vi "Write Timings Header.vi"(8 "error in (no error)":errorcluster, 11 "Save Image in":refnum<class "Save Image.lvclass">) -> (0 "error out":errorcluster, 3 "Save Image out":refnum<class "Save Image.lvclass">)   [LabVIEW 2018, in "Save Image.lvclass"]
uses:
  Save Image.lvclass
  <userlib>/gfitsio/gfitsio-write-key-string.vi
  <userlib>/gfitsio/gfitsio.lvlib
  Simulated_Header/Simulated_Header.lvclass
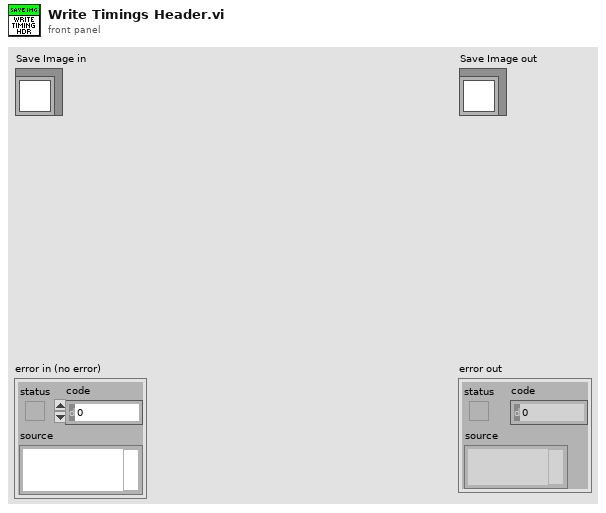
[diagram p1: front panel]
types:
  T1 = typedef "gfitsio.lvlib/gfitsio-refnum.ctl" = refnum<k1>
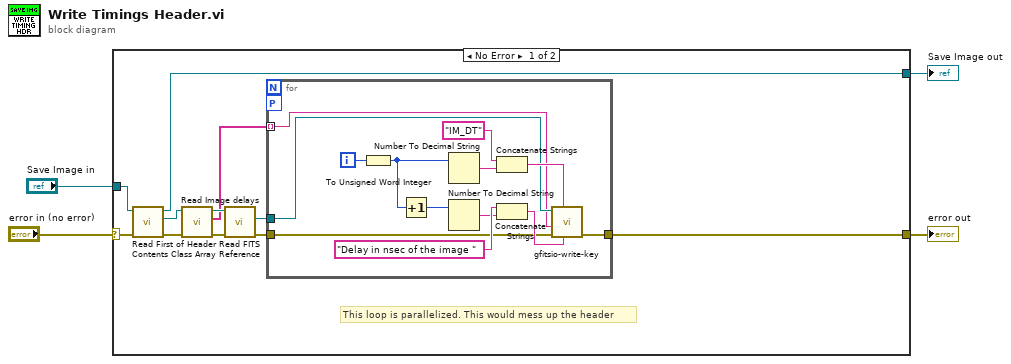
[diagram p0: block diagram]
diagram:
  n1 = case shown="No Error" "error in (no error)" {
    selector: "error in (no error)" -> [w11 w30]
    tunnel: [w15 w30] -> w3
    tunnel: [w5 w29] -> w1
    tunnel: "Save Image in" -> [w13 w29]
    frame No Error {
      # "This loop is parallelized. This would mess up the header"
      n2 = call "Read First of Header Contents Class Array.vi"("error in (no error)"=w11, "Save Image in"=w13) -> ("error out"=w12:errorcluster, "Simulated_Header.lvclass"=w14:refnum<class "Simulated_Header.lvclass">, "Save Image out"=w5:refnum<class "Save Image.lvclass">)  [unwired: 7 in]
      n3 = call "Read Image delays.vi"("error in (no error)"=w12, "Header in"=w14) -> ("error out"=w9:errorcluster, "Image delays"=w7:string[], "Header out"=w10:refnum<class "Simulated_Header.lvclass">)  [unwired: 7 in]
      n4 = call "Read FITS Reference.vi"("error in (no error)"=w9, "Simulated_Header in"=w10) -> ("error out"=w6:errorcluster, "gfits refnum"=w8:T1)  [unwired: 7 in, 1 out]
      n5 = for {
        tunnel: [w23] -> w15
        workers-P: _ -> [_]
        tunnel: w8 -> [w18]
        tunnel: w7 -> [w17] mode=indexing
        tunnel: w6 -> [w16]
        i -> [w19]
        n6 = To Unsigned Word Integer(number=w19) -> (unsigned 16bit integer=w20:u16)
        n7 = Increment(x=w20) -> (x+1=w25:u16)
        n8 = Number To Decimal String(number=w20) -> (decimal integer string=w27:string)  [unwired: 1 in]
        n9 = Number To Decimal String(number=w25) -> (decimal integer string=w21:string)  [unwired: 1 in]
        n10 = Concatenate Strings("IM_DT", w27) -> (w26:string)
        n11 = Concatenate Strings("Delay in nsec of the image " ("comment"), w21) -> (w24:string)
        n12 = call-poly <userlib>:"gfitsio-write-key.vi"("comment"=w24, "keyname"=w26, "error in (no error)"=w16, "value"=w17, "gfits refnum"=w18) -> ("error out"=w23:errorcluster)  [unwired: 5 in, 1 out]
      }
    }
    frame Error {
    }
  }
  "error out" <- w3
  "Save Image out" <- w1
